vi "Configure PRACH Power Result Enabled.vi"(7 "Power Vs Preamble (Off)":bool, 8 "error in (no error)":errorcluster, 9 "Power Dynamics (On)":bool=TRUE, 10 "Instance (1)":T1=1, 11 "VISA resource name":refnum<visa-resource-name>) -> (0 "error out":errorcluster, 3 "VISA resource name out":refnum<visa-resource-name>)   [LabVIEW 2020, in "Rohde&Schwarz CMWXP NR FR1 Measurement.lvlib"]
doc: "Enables or disables the evaluation of results in the PRACH Power Dynamics measurement.\n\nAttributes:\nRSCMWXPNRFR1M_ATTR_PRACH_POWER_DYNAMICS_RESULT_ENABLED\nRSCMWXPNRFR1M_ATTR_PRACH_POWER_VS_PREAMBLE_RESULT_ENABLED\n\nRemote-control commands:\nCONFigure:NRSub:MEAS<i>:PRACh:RESult:PDYNamics\nCONFigure:NRSub:MEAS<i>:PRACh:RESult:PVPReamble"
uses:
  <instrlib>/Rohde&Schwarz CMWXP NR FR1 Measurement/Rohde&Schwarz CMWXP NR FR1 Measurement.lvlib
  <instrlib>/Rohde&Schwarz CMWXP NR FR1 Measurement/Private/_Instance.ctl
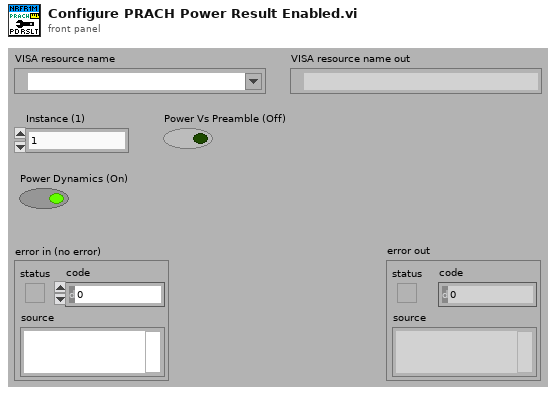
[diagram p1: front panel]
types:
  T1 = typedef "Rohde&Schwarz CMWXP NR FR1 Measurement.lvlib/_Instance.ctl" = i32
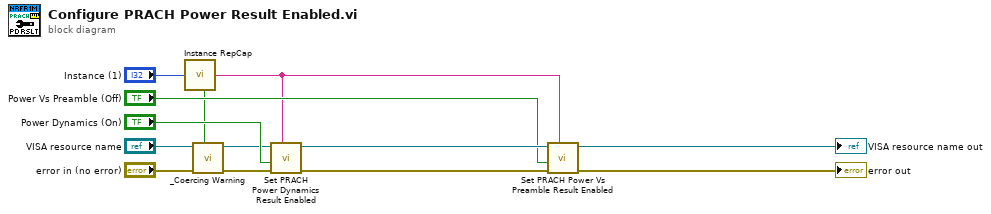
[diagram p0: block diagram]
diagram:
  n1 = call <instrlib>:"Instance RepCap.vi"("Instance In"="Instance (1)") -> ("In Range?"=w2:bool, "RepCap Identifier Out"=w1:string)  [unwired: 1 in]
  n2 = call <instrlib>:"_Coercing Warning.vi"("In Range?"=w2, "error in (no error)"="error in (no error)", "VISA resource name"="VISA resource name") -> ("error out"=w5:errorcluster, "VISA resource name out"=w4:refnum<visa-resource-name>)  [unwired: 7 in]
  n3 = call "Set PRACH Power Dynamics Result Enabled"("Repeated Capabilities"=w1, "error in (no error)"=w5, "PRACH Power Dynamics Result Enabled (OFF)"="Power Dynamics (On)", "instrument handle"=w4) -> ("error out"=w9:errorcluster, "instrument handle out"=w10:refnum<visa-resource-name>)  [unwired: 6 in]
  n4 = call "Set PRACH Power Vs Preamble Result Enabled"("Repeated Capabilities"=w1, "error in (no error)"=w9, "PRACH Power Vs Preamble Result Enabled (OFF)"="Power Vs Preamble (Off)", "instrument handle"=w10) -> ("error out"=→"error out":errorcluster, "instrument handle out"=→"VISA resource name out":refnum<visa-resource-name>)  [unwired: 6 in]
